vi "PLC.CheckStatus.vi"(7 "Idx":i32, 8 "error in":errorcluster, 10 "Slot":i32, 11 "Data_in":T1={"Status"={"Idx"=0, "ConnRef"=0, "State"=enum."Off", "LiveBitTimer"=timestamp(0 s since 1904-01-01)}, "Sets"={"Enable"=FALSE, "IP"="", "Rack"=0, "Slot"=0, "LifeBitTimer_s"=0.0, "DataBlockAddr_PCStatus"=0, "DataBlockAddr_PLCStatus"=1, "DataBlockAddr_PLCNewData"=[], "DataBlockSize_PLCNewData"=[], "DataBlockAddr_PLCChangeOver"=[], "DataBlockSize_PLCChangeOver"=[], "DataBlockAddr_PCChangeOver"=[], "DataBlockAddr_PLCCheckStatus"=[], "DataBlockSize_PLCCheckStatus"=[], "DataBlockAddr_PCCheckStatus"=[]}, "PCstatus"={"General"={"LifeBit"=FALSE, "DbRun"=FALSE}, "Stations"=[]}, "PLCstatus"={"General"={"LifeBit"=FALSE}, "Stations"=[]}}) -> (0 "error out":errorcluster, 3 "Data_out":T1={"Status"={"Idx"=0, "ConnRef"=0, "State"=enum."Off", "LiveBitTimer"=timestamp(0 s since 1904-01-01)}, "Sets"={"Enable"=FALSE, "IP"="", "Rack"=0, "Slot"=0, "LifeBitTimer_s"=0.0, "DataBlockAddr_PCStatus"=0, "DataBlockAddr_PLCStatus"=1, "DataBlockAddr_PLCNewData"=[], "DataBlockSize_PLCNewData"=[], "DataBlockAddr_PLCChangeOver"=[], "DataBlockSize_PLCChangeOver"=[], "DataBlockAddr_PCChangeOver"=[], "DataBlockAddr_PLCCheckStatus"=[], "DataBlockSize_PLCCheckStatus"=[], "DataBlockAddr_PCCheckStatus"=[]}, "PCstatus"={"General"={"LifeBit"=FALSE, "DbRun"=FALSE}, "Stations"=[]}, "PLCstatus"={"General"={"LifeBit"=FALSE}, "Stations"=[]}})   [LabVIEW 2016]
doc: "Get test results (measurement values) from PLC and save to database\n\nWabco 2017 All right reserved\nAuthor: maciej.szupienko@wabco-auto.com"
uses:
  PLC.Data.ctl
  PLC.Data.Status.ctl
  PLC.State.ctl
  PLC.Data.Sets.ctl
  LowLevel/PLC.DataBlock.PCstatus.ctl
  LowLevel/PLC.DataBlock.PCstatus.General.ctl
  LowLevel/PLC.DataBlock.PCstatus.Station.ctl
  LowLevel/PLC.DataBlock.PLCstatus.ctl
  LowLevel/PLC.DataBlock.PLCstatus.General.ctl
  LowLevel/PLC.DataBlock.PLCstatus.Station.ctl
  LowLevel/PLC.DataBlock.PLCcheckstatus.ctl
  LowLevel/PLC.DataBlock.PCcheckstatus.ctl
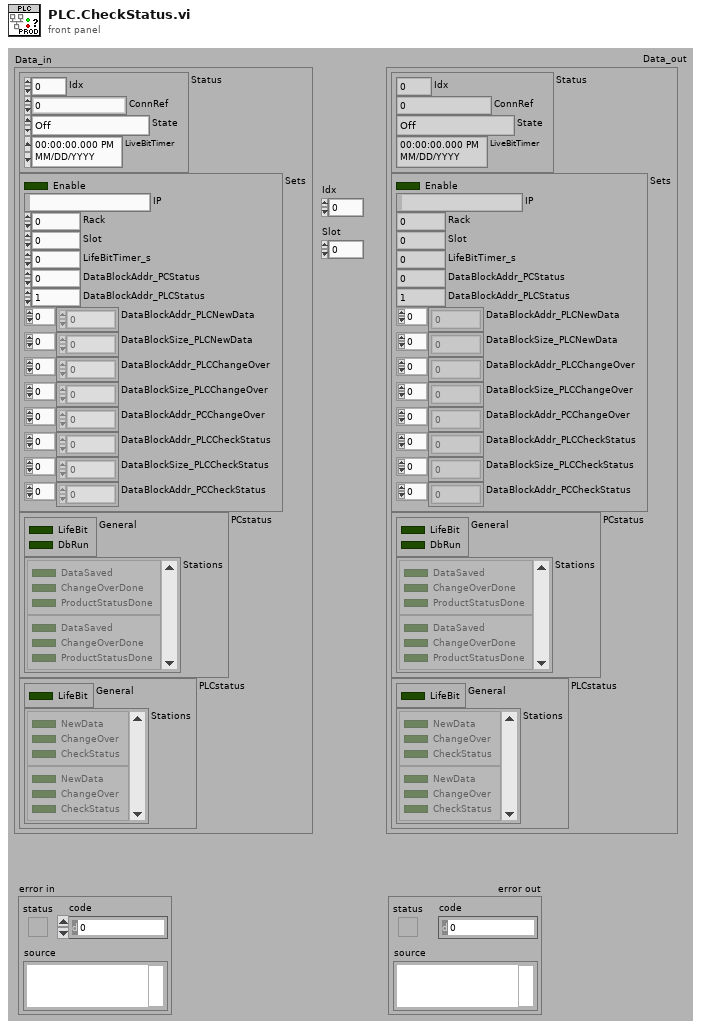
[diagram p1: front panel]
types:
  T1 = typedef "PLC.Data.ctl" = cluster{"Status":T2, "Sets":T4, "PCstatus":T5, "PLCstatus":T8}
  T2 = typedef "PLC.Data.Status.ctl" = cluster{"Idx":i32, "ConnRef":u64, "State":T3, "LiveBitTimer":timestamp}
  T3 = typedef "PLC.State.ctl" = enum32{"Off", "Error", "Idle", "Run"}
  T4 = typedef "PLC.Data.Sets.ctl" = cluster{"Enable":bool, "IP":string, "Rack":i32, "Slot":i32, "LifeBitTimer_s":dbl, "DataBlockAddr_PCStatus":i32, "DataBlockAddr_PLCStatus":i32, "DataBlockAddr_PLCNewData":i32[], "DataBlockSize_PLCNewData":i32[], "DataBlockAddr_PLCChangeOver":i32[], "DataBlockSize_PLCChangeOver":i32[], "DataBlockAddr_PCChangeOver":i32[], "DataBlockAddr_PLCCheckStatus":i32[], "DataBlockSize_PLCCheckStatus":i32[], "DataBlockAddr_PCCheckStatus":i32[]}
  T5 = typedef "PLC.DataBlock.PCstatus.ctl" = cluster{"General":T6, "Stations":T7[]}
  T6 = typedef "PLC.DataBlock.PCstatus.General.ctl" = cluster{"LifeBit":bool, "DbRun":bool}
  T7 = typedef "PLC.DataBlock.PCstatus.Station.ctl" = cluster{"DataSaved":bool, "ChangeOverDone":bool, "ProductStatusDone":bool}
  T8 = typedef "PLC.DataBlock.PLCstatus.ctl" = cluster{"General":T9, "Stations":T10[]}
  T9 = typedef "PLC.DataBlock.PLCstatus.General.ctl" = cluster{"LifeBit":bool}
  T10 = typedef "PLC.DataBlock.PLCstatus.Station.ctl" = cluster{"NewData":bool, "ChangeOver":bool, "CheckStatus":bool}
  T11 = typedef "PLC.DataBlock.PCcheckstatus.ctl" = cluster{"Ref":string, "Serial":string, "StatusPrev":i8, "StatusThis":i8, "Repetitions":u8}
  T12 = typedef "PLC.DataBlock.PLCcheckstatus.ctl" = cluster{"Ref1":string, "Serial1":string, "Ref2":string, "Serial2":string}
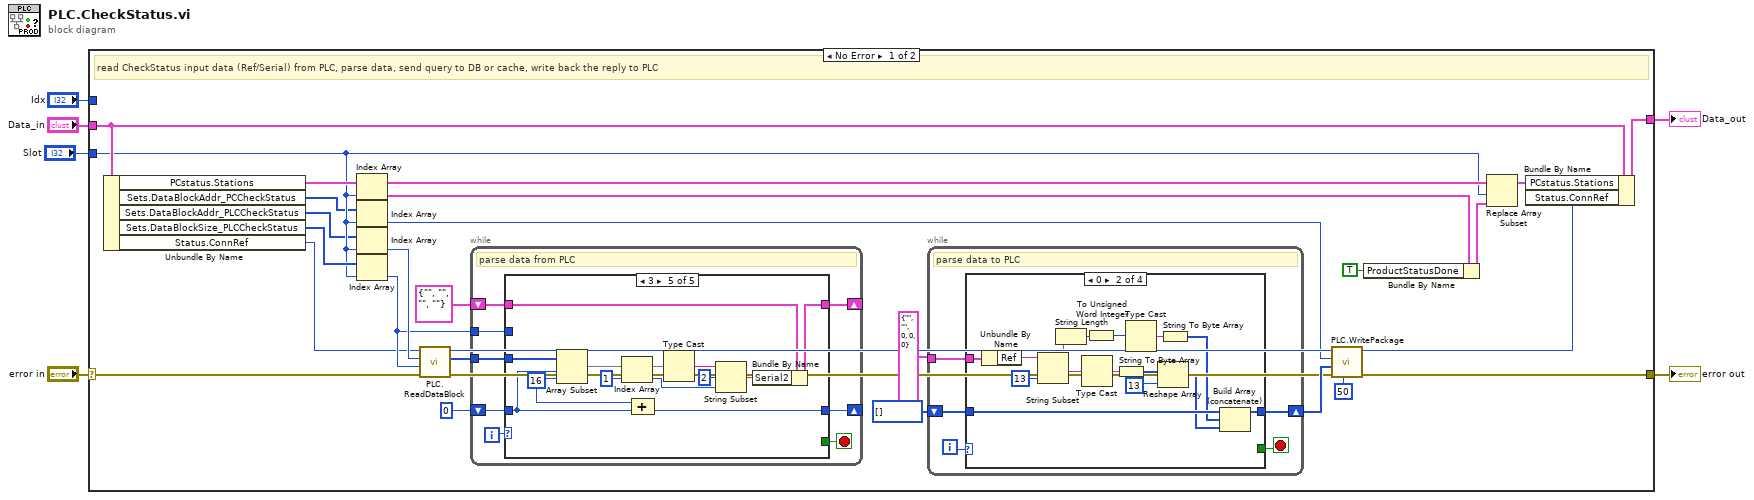
[diagram p0: block diagram]
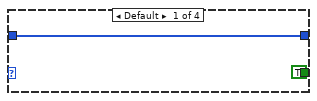
[diagram p2: hidden frame]
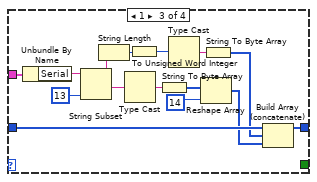
[diagram p3: hidden frame]
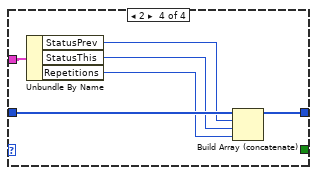
[diagram p4: hidden frame]
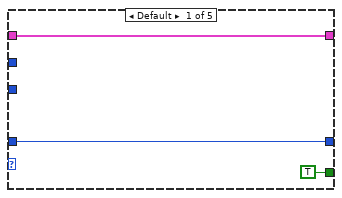
[diagram p5: hidden frame]
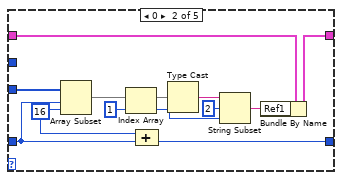
[diagram p6: hidden frame]
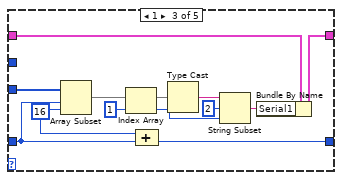
[diagram p7: hidden frame]
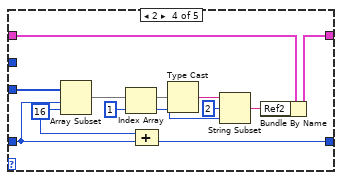
[diagram p8: hidden frame]
diagram:
  n1 = case shown="No Error" "error in" {
    selector: "error in" -> [w32 w135]
    tunnel: [w20 w135] -> w3
    tunnel: "Data_in" -> [w30 w134]
    tunnel: [w33 w134] -> w5
    tunnel: "Idx" -> [_ _]
    tunnel: "Slot" -> [w15 _]
    frame No Error {
      # "read CheckStatus input data (Ref/Serial) from PLC, parse data, send query to DB or cache, write back the reply to PLC"
      n2 = Unbundle By Name(w30) -> ("PCstatus.Stations"=w16:T7[], "Sets.DataBlockAddr_PCCheckStatus"=w11:i32[], "Sets.DataBlockAddr_PLCCheckStatus"=w12:i32[], "Sets.DataBlockSize_PLCCheckStatus"=w22:i32[], "Status.ConnRef"=w10:u64)
      n3 = Index Array(array=w16, index=w15) -> (element=w28:T7)
      n4 = Index Array(array=w11, index=w15) -> (element=w13:i32)
      n5 = Index Array(array=w12, index=w15) -> (element=w31:i32)
      n6 = Index Array(array=w22, index=w15) -> (element=w23:i32)
      n7 = call "PLC.ReadDataBlock.vi"("error in (no error)"=w32, "Amount (1)"=w23, "Block"=w31, "Ref"=w10) -> ("error out"=w8:errorcluster, "data out"=w26:u8[], "ref out"=w21:u64)  [unwired: 5 in]
      n8 = while {
        tunnel: w26 -> [w77]
        shift-right: [w80] -> _
        shift-left: 0 -> [w81]
        shift-right: [w79] -> _
        shift-left: T12 {"Ref1"="", "Serial1"="", "Ref2"="", "Serial2"=""} ("element") -> [w78]
        tunnel: w23 -> [w76]
        i -> [w82]
        stop <- w75 stop-if-true
        # "parse data from PLC"
        n9 = case shown="3" w82 {
          tunnel: w81 -> [w84 w88 w100 w112 w124]
          tunnel: [w84 w87 w99 w111 w123] -> w80
          tunnel: [w85 w97 w109 w121 w133] -> w79
          tunnel: w78 -> [w85 w96 w108 w120 w132]
          tunnel: w77 -> [_ w91 w103 w115 w127]
          tunnel: w76 -> [_ _ _ _ _]
          tunnel: [TRUE _ _ _ _] -> w75
          frame Default {
          }
          frame 0 {
            w89 = 16 ("length")
            n10 = Array Subset(array=w91, index=w88, length=w89) -> (w93:u8[])
            n11 = Index Array(array=w93, index=1) -> (element=w86:u8)
            n12 = Compound Arithmetic op=ADD(w89, w88) -> (w87:i32)
            n13 = Type Cast(x=w93) -> (*(type *) &x=w92:string)  [unwired: 1 in]
            n14 = String Subset(string=w92, offset (0)=2, length (rest)=w86) -> (substring=w90:string)
            n15 = Bundle By Name(cluster=w96, "Ref1"=w90) -> (w97:T12)
          }
          frame 1 {
            w101 = 16 ("length")
            n16 = Array Subset(array=w103, index=w100, length=w101) -> (w105:u8[])
            n17 = Index Array(array=w105, index=1) -> (element=w98:u8)
            n18 = Compound Arithmetic op=ADD(w101, w100) -> (w99:i32)
            n19 = Type Cast(x=w105) -> (*(type *) &x=w104:string)  [unwired: 1 in]
            n20 = String Subset(string=w104, offset (0)=2, length (rest)=w98) -> (substring=w102:string)
            n21 = Bundle By Name(cluster=w108, "Serial1"=w102) -> (w109:T12)
          }
          frame 2 {
            w113 = 16 ("length")
            n22 = Array Subset(array=w115, index=w112, length=w113) -> (w117:u8[])
            n23 = Index Array(array=w117, index=1) -> (element=w110:u8)
            n24 = Compound Arithmetic op=ADD(w113, w112) -> (w111:i32)
            n25 = Type Cast(x=w117) -> (*(type *) &x=w116:string)  [unwired: 1 in]
            n26 = String Subset(string=w116, offset (0)=2, length (rest)=w110) -> (substring=w114:string)
            n27 = Bundle By Name(cluster=w120, "Ref2"=w114) -> (w121:T12)
          }
          frame 3 {
            w125 = 16 ("length")
            n28 = Array Subset(array=w127, index=w124, length=w125) -> (w129:u8[])
            n29 = Index Array(array=w129, index=1) -> (element=w122:u8)
            n30 = Compound Arithmetic op=ADD(w125, w124) -> (w123:i32)
            n31 = Type Cast(x=w129) -> (*(type *) &x=w128:string)  [unwired: 1 in]
            n32 = String Subset(string=w128, offset (0)=2, length (rest)=w122) -> (substring=w126:string)
            n33 = Bundle By Name(cluster=w132, "Serial2"=w126) -> (w133:T12)
          }
        }
      }
      n34 = while {
        tunnel: T11 {"Ref"="", "Serial"="", "StatusPrev"=0, "StatusThis"=0, "Repetitions"=0} ("PCcheckstatus") -> [w37]
        shift-right: [w35] -> w18
        shift-left: u8[] [] ("data in") -> [w34]
        i -> [w38]
        stop <- w36 stop-if-true
        # "parse data to PLC"
        n35 = case shown="0" w38 {
          tunnel: w37 -> [_ w54 w68 w74]
          tunnel: [TRUE _ _ _] -> w36
          tunnel: [w39 w53 w67 w69] -> w35
          tunnel: w34 -> [w39 w52 w66 w73]
          frame Default {
          }
          frame 0 {
            n36 = Unbundle By Name(w54) -> ("Ref"=w50:string)
            n37 = String Subset(string=w50, length (rest)=13 ("length (rest)")) -> (substring=w45:string)  [unwired: 1 in]
            n38 = String Length(string=w45) -> (length=w51:i32)
            n39 = Type Cast(x=w45) -> (*(type *) &x=w46:string)  [unwired: 1 in]
            n40 = To Unsigned Word Integer(number=w51) -> (unsigned 16bit integer=w49:u16)
            n41 = String To Byte Array(string=w46) -> (unsigned byte array=w44:u8[])
            n42 = Type Cast(x=w49) -> (*(type *) &x=w48:string)  [unwired: 1 in]
            n43 = Reshape Array(w44, 13 ("length (rest)")) -> (w43:u8[])
            n44 = String To Byte Array(string=w48) -> (unsigned byte array=w47:u8[])
            n45 = Build Array (concatenate)(w52, w47, w43) -> (w53:u8[])
          }
          frame 1 {
            n46 = Unbundle By Name(w68) -> ("Serial"=w64:string)
            n47 = String Subset(string=w64, length (rest)=13 ("length (rest)")) -> (substring=w59:string)  [unwired: 1 in]
            n48 = String Length(string=w59) -> (length=w65:i32)
            n49 = Type Cast(x=w59) -> (*(type *) &x=w60:string)  [unwired: 1 in]
            n50 = To Unsigned Word Integer(number=w65) -> (unsigned 16bit integer=w63:u16)
            n51 = String To Byte Array(string=w60) -> (unsigned byte array=w58:u8[])
            n52 = Type Cast(x=w63) -> (*(type *) &x=w62:string)  [unwired: 1 in]
            n53 = Reshape Array(w58, 14 ("length (rest)")) -> (w57:u8[])
            n54 = String To Byte Array(string=w62) -> (unsigned byte array=w61:u8[])
            n55 = Build Array (concatenate)(w66, w61, w57) -> (w67:u8[])
          }
          frame 2 {
            n56 = Unbundle By Name(w74) -> ("StatusPrev"=w72:i8, "StatusThis"=w71:i8, "Repetitions"=w70:u8)
            n57 = Build Array (concatenate)(w73, w72, w71, w70) -> (w69:u8[])
          }
        }
      }
      n58 = call "PLC.WritePackage.vi"("max package size  (0: full)"=50, "error in (no error)"=w8, "data"=w18, "addr"=w13, "Ref in"=w21) -> ("error out"=w20:errorcluster, "Ref out"=w17:u64)  [unwired: 5 in]
      n59 = Bundle By Name(cluster=w28, "ProductStatusDone"=TRUE ("ChangeOverDone")) -> (w27:T7)
      n60 = Replace Array Subset(array=w16, new element=w27, index=w15) -> (w29:T7[])
      n61 = Bundle By Name(cluster=w30, "PCstatus.Stations"=w29, "Status.ConnRef"=w17) -> (w33:T1)
    }
    frame Error {
    }
  }
  "error out" <- w3
  "Data_out" <- w5
